vi "Select Graph Channels.vi"(8 "error in (no error)":errorcluster, 9 "Y Group Channels":string[][](array[string]), 10 "X Group Channels":string[][](array[string]), 11 "Common Measurements in":refnum<class "Common Measurements.lvclass">) -> (0 "error out":errorcluster, 3 "Common Measurements out":refnum<class "Common Measurements.lvclass">)   [LabVIEW 2015, in "Common Measurements.lvclass"]
uses:
  Common Measurements.lvclass
  Mag Lab Measure Base/Mag Lab Measure Base.lvclass/Mag Lab Measure Base.ctl
  Common Measurements.lvclass/Common Measurements.ctl
  MagLabGraph Messages/Add file Msg/Add file Msg.lvclass/Add file Msg.ctl
  <vilib>/ActorFramework/Message Enqueuer/Message Enqueuer.lvclass/Message Enqueuer.ctl
  MagLabGraph Messages/Select File Group Channel Msg/Select File Group Channel Msg.lvclass/Select File Group Channel Msg.ctl
  <vilib>/ActorFramework/Message Enqueuer/Enqueue.vi
  <vilib>/ActorFramework/Message Priority Queue/Priority Enqueue.vi
  Mag Lab Error Handler/Send Error.vi
  <vilib>/ActorFramework/Message Enqueuer/Message Enqueuer.lvclass
  MagLabGraph Messages/Add file Msg/Add file Msg.lvclass
  MagLabGraph Messages/Select File Group Channel Msg/Select File Group Channel Msg.lvclass
  Mag Lab Measure Base/Mag Lab Measure Base.lvclass
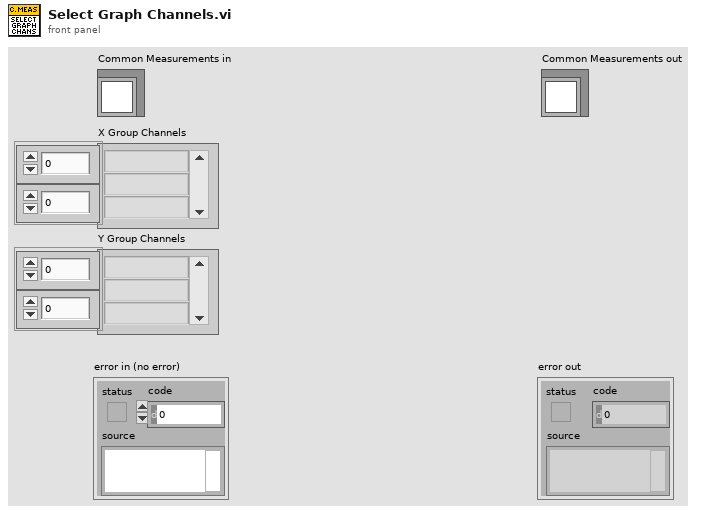
[diagram p1: front panel]
types:
  T1 = typedef "File_Group_Chan_Abbr.ctl" = cluster{"File Path Control":path, "Group":string, "Channel":string, "Abbreviated":string}
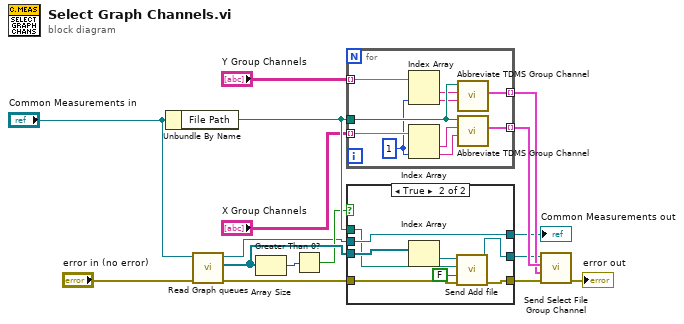
[diagram p0: block diagram]
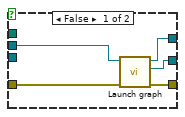
[diagram p2: hidden frame]
diagram:
  n1 = Unbundle By Name("Common Measurements in") -> ("File Path"=w12:path)
  n2 = call "Read Graph queues.vi"("error in (no error)"="error in (no error)", "Mag Lab Measure Base in"="Common Measurements in") -> ("error out"=w13:errorcluster, "Graph queues"=w15:refnum<class "Message Enqueuer.lvclass">[], "Mag Lab Measure Base out"=w2:refnum<class "Common Measurements.lvclass">)  [unwired: 7 in]
  n3 = Array Size(array=w15) -> (size(s)=w4:i32)
  n4 = Greater Than 0?(x=w4) -> (x > 0?=w3:bool)
  n5 = for {
    tunnel: w12 -> [w26]
    tunnel: "X Group Channels" -> [w25] mode=indexing
    tunnel: "Y Group Channels" -> [w24] mode=indexing
    tunnel: [w18] -> w9 mode=indexing
    tunnel: [w17] -> w8 mode=indexing
    w23 = 1 ("index")
    n6 = Index Array(array=w24, index #2=w23) -> (element #1=w20:string, element #2=w19:string)  [unwired: 1 in]
    n7 = Index Array(array=w25, index #2=w23) -> (element #1=w22:string, element #2=w21:string)  [unwired: 1 in]
    n8 = call "Abbreviate TDMS Group Channel.vi"("Channel"=w19, "Group"=w20, "File Path Control"=w26) -> ("Cluster"=w17:T1)  [unwired: 7 in, 1 out]
    n9 = call "Abbreviate TDMS Group Channel.vi"("Channel"=w21, "Group"=w22, "File Path Control"=w26) -> ("Cluster"=w18:T1)  [unwired: 7 in, 1 out]
  }
  n10 = case shown="True" w3 {
    tunnel: w15 -> [_ w39]
    tunnel: w13 -> [w27 w35]
    tunnel: w12 -> [_ w36]
    tunnel: [w29 w33] -> w7
    tunnel: [w28 w34] -> w6
    tunnel: w2 -> [w31 w38]
    tunnel: [w30 w38] -> w1
    frame False {
      n11 = call-dynamic "Launch graph.vi"("error in (no error)"=w27, "Common Measurements in"=w31) -> ("error out"=w28:errorcluster, "Message Enqueuer out"=w29:refnum<class "Message Enqueuer.lvclass">, "Common Measurements out"=w30:refnum<class "Common Measurements.lvclass">)  [unwired: 7 in]
    }
    frame True {
      n12 = Index Array(array=w39) -> (element=w37:refnum<class "Message Enqueuer.lvclass">)  [unwired: 1 in]
      n13 = call "Send Add file.vi"("error in (no error)"=w35, "Insert in front"=FALSE, "File Path Control"=w36, "Message Enqueuer"=w37) -> ("error out"=w34:errorcluster, "Message Enqueuer out"=w33:refnum<class "Message Enqueuer.lvclass">)  [unwired: 6 in]
    }
  }
  "Common Measurements out" <- w1
  n14 = call "Send Select File Group Channel.vi"("error in (no error)"=w6, "File-group-channel Y"=w8, "File-group-channel X"=w9, "Message Enqueuer"=w7) -> ("error out"=→"error out":errorcluster)  [unwired: 6 in, 1 out]
